vi "GUI_HPD ESP.vi"() -> ()   [LabVIEW 2013]
uses:
  shared programs/GUI_Template/GUI_master/tcp_new_data_event.ctl
  shared programs/GUI_Template/GUI_master/tcp new data cluster.ctl
  <vilib>/vision/Image Controls.llb/IMAQ Image.ctl
panel:
  in  "position.axis 1::3":dbl caption="ESP Axis 1" min=-6.0 max=6.0
  in  "position.axis 2::3":dbl caption="ESP Axis 2" min=-6.0 max=6.0
  in  "position.axis 2::2":dbl caption="ESP Axis 2" min=-6.0 max=6.0
  in  "position.axis 1::2":dbl caption="ESP Axis 1" min=-6.0 max=6.0
  in  "stepsize::3":dbl caption="Step Size" min=0.0 max=1.0
  in  "stepsize::2":dbl caption="Step Size" min=0.0 max=1.0
  in  "GUIdevice 3":string="HPD_ESP2"
  in  "GUIdevice 2":string="HPD_ESP1"
  in  "relativeMove.Axis 1neg::3":bool caption="Right"
  in  "relativeMove.Axis 1pos::3":bool caption="Left"
  in  "relativeMove.Axis 2pos::3":bool caption="Down"
  in  "relativeMove.Axis 2neg::3":bool caption="relativemove.Axis 3neg::6"
  in  "relativeMove.Axis 1neg::2":bool
  in  "relativeMove.Axis 1pos::2":bool
  in  "relativeMove.Axis 2pos::2":bool
  in  "relativeMove.Axis 2neg::2":bool
  out "image::1":T1(plugin-control) caption="HPD CCD CAM"
  in  "exposure::1":dbl=0.001 caption="Exposure" min=3.8e-05 max=1.0 format="%_4p"
  in  "insert tag":bool=TRUE
  in  "stop":bool
  in  "trigger::1":bool caption="Trigger"
  in  "GUIdevice 1":string="HPD_CCD"
  out "tcp data event":T2
  out "error IO 2":errorcluster
  # "HPD_ESP1"
  # "HPD_ESP2"
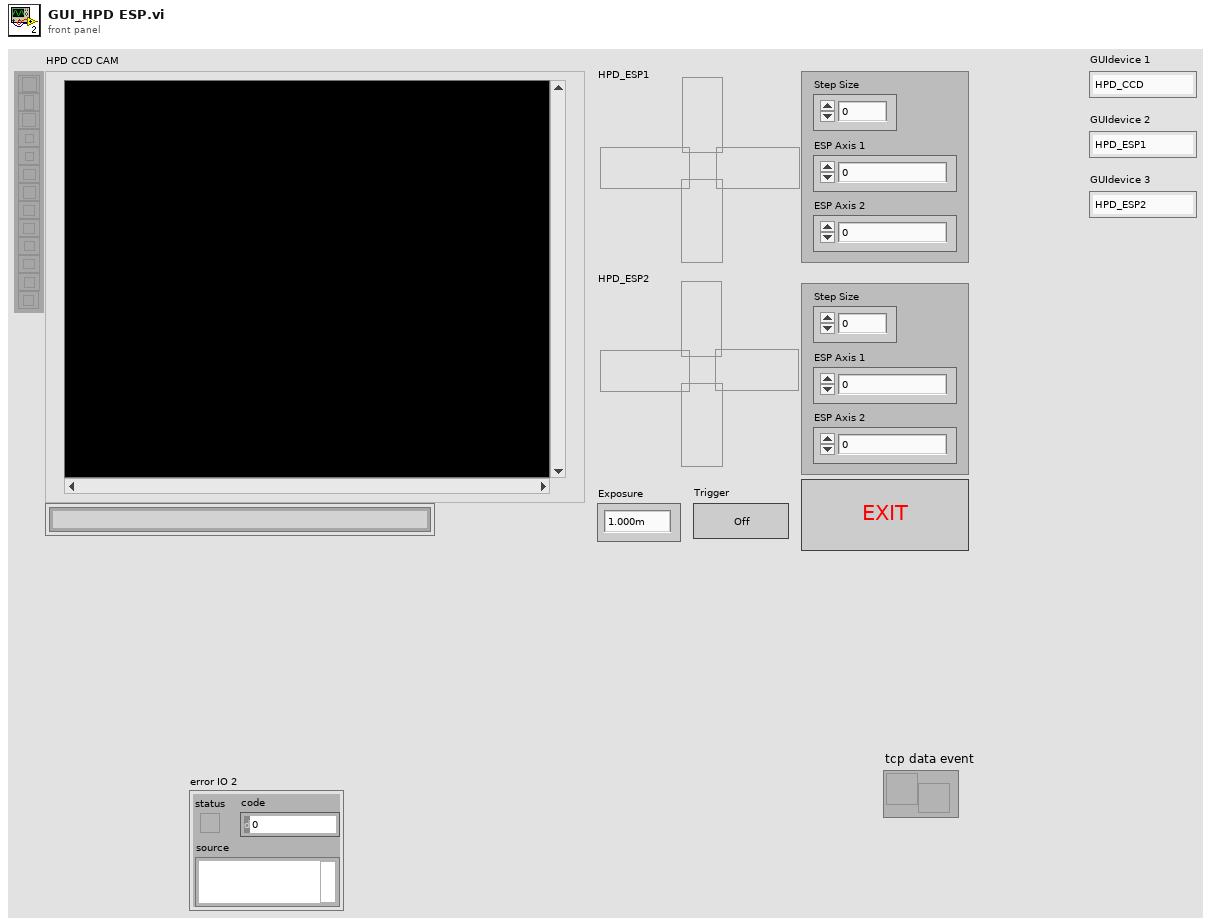
[diagram p1: front panel]
types:
  T1 = typedef "IMAQ Image.ctl" = refnum<image>
  T2 = typedef "tcp_new_data_event.ctl" = refnum<user-event>
  T3 = typedef "tcp new data cluster.ctl" = cluster{"EventEnum":enum16{"new data", "connection status update"}, "Device name":string}
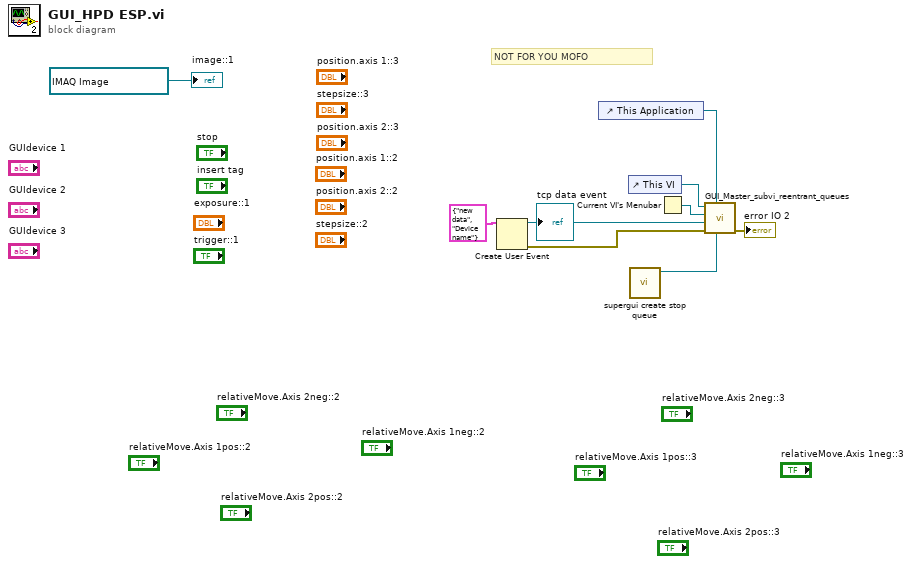
[diagram p0: block diagram]
diagram:
  # "NOT FOR YOU MOFO"
  n1 = Create User Event(user event datatype=T3 {"EventEnum"=enum."new data", "Device name"="Device name"} ("New Event")) -> (user event=w4:refnum<user-event>, error out=w5:errorcluster)  [unwired: 1 in]
  "tcp data event" <- w4
  n2 = control-ref of="This Application"() -> (w2:refnum<vi>)
  n3 = control-ref of="This VI"() -> (w8:refnum<vi>)
  n4 = call "supergui create stop queue.vi"() -> ("STOP Queue out"=w1:refnum<queue>)  [unwired: 11 in]
  n5 = Current VI's Menubar() -> (w7:refnum<k9>)
  n6 = call "GUI_Master_subvi_reentrant_queues.vi"("STOP Queue in"=w1, "This Application"=w2, "error in (no error)"=w5, "tcp data event"=w4, "Caller menu reference"=w7, "Caller VI ref"=w8) -> ("error out"=→"error IO 2":errorcluster)  [unwired: 5 in]
  "image::1" <- T1 refnum ("New Image")
